vi "Keithley Sweep and Acquire Measurements.vi"(4 "Source Delay (s)":dbl=0.1, 5 "Sweep Direction":u16(ring) items=["Low to high", "High to low"], 6 "Number of Points":u32=5, 7 "Maximum Amplitude":dbl=2.0, 8 "Minimum Amplitude":dbl=1.0, 9 "VISA resource name":refnum<visa-resource-name>) -> (0 "Measurement Complete":bool, 2 "Data Array":dbl[][](array[numeric]), 3 "VISA resource name out":refnum<visa-resource-name>)   [LabVIEW 2011]
doc: "Configures a sweep and takes voltage and current readings at each point."
uses:
  <instrlib>/Keithley 24XX/Public/Data/Read (Multiple Points).vi
  <instrlib>/Keithley 24XX/Keithley 24XX.lvlib
panel:
  in  "Source Mode  (0: Voltage)":u16(ring) items=["Voltage", "Current"]
  in  "Timeout (10000 ms)":i32=60000 format="%#.6g"
  in  "Compliance  Level":dbl=0.1
  # "(c) 2006 National Instruments.  ALL RIGHTS RESERVED."
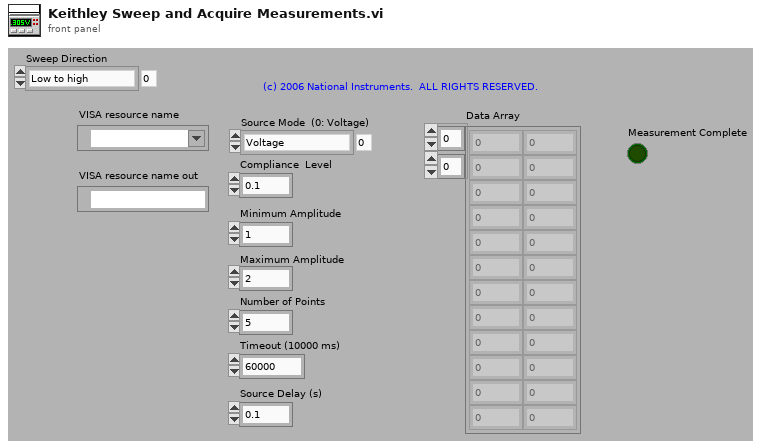
[diagram p1: front panel]
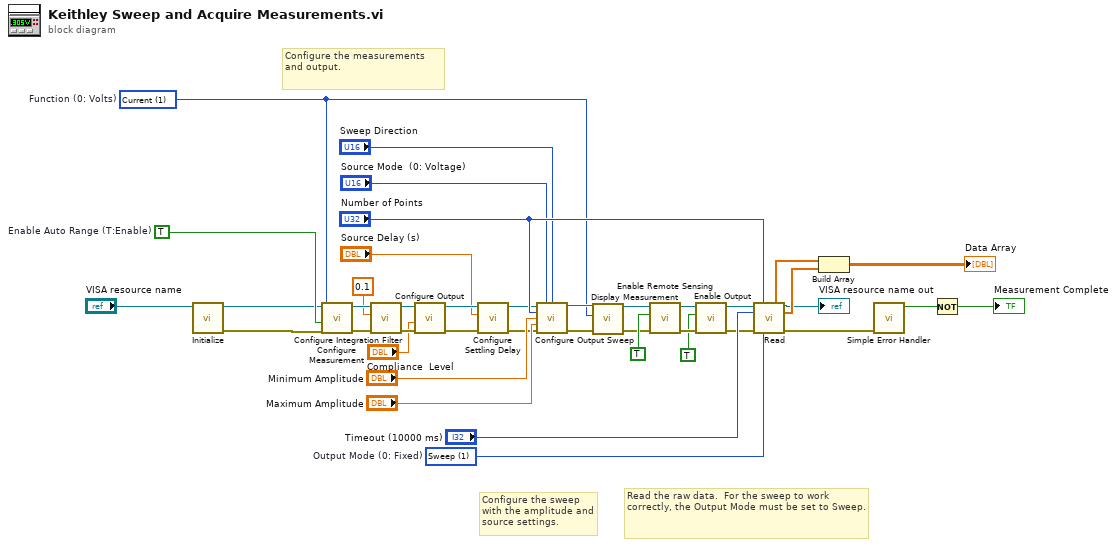
[diagram p0: block diagram]
diagram:
  w30 = TRUE  # Enable Auto Range (T:Enable)
  w12 = u16 1 items=["Volts", "Current", "Resistance"]  # Function (0: Volts)
  w33 = u16 1 items=["Fixed", "Sweep", "List"]  # Output Mode (0: Fixed)
  # "Read the raw data.  For the sweep to work correctly, the Output Mode must be set to Sweep."
  # "Configure the sweep with the amplitude and source settings."
  # "Configure the measurements and output."
  n1 = call <instrlib>:"Initialize.vi"("VISA resource name"="VISA resource name") -> ("error out"=w10:errorcluster, "VISA resource name out"=w11:refnum<visa-resource-name>)  [unwired: 9 in]
  n2 = call <instrlib>:"Configure Measurement.vi"("error in (no error)"=w10, "Enable Auto Range (T:Enable)"=w30, "Function (0: Volts)"=w12, "VISA resource name"=w11) -> ("error out"=w17:errorcluster, "VISA resource name out"=w18:refnum<visa-resource-name>)  [unwired: 6 in]
  n3 = call <instrlib>:"Configure Integration Filter.vi"("error in (no error)"=w17, "Measurement Speed (1 PLC)"=0.1, "VISA resource name"=w18) -> ("error out"=w8:errorcluster, "VISA resource name out"=w9:refnum<visa-resource-name>)  [unwired: 7 in]
  n4 = call <instrlib>:"Configure Output.vi"("error in (no error)"=w8, "Compliance  Level (0.1)"="Compliance  Level", "VISA resource name"=w9) -> ("error out"=w4:errorcluster, "VISA resource name out"=w5:refnum<visa-resource-name>)  [unwired: 7 in]
  n5 = call <instrlib>:"Configure Settling Delay.vi"("error in (no error)"=w4, "Manual Settling Delay (0 sec)"="Source Delay (s)", "VISA resource name"=w5) -> ("error out"=w2:errorcluster, "VISA resource name out"=w3:refnum<visa-resource-name>)  [unwired: 7 in]
  n6 = call <instrlib>:"Configure Output Sweep.vi"("VISA resource name"=w3, "Source Mode  (0: Voltage)"="Source Mode  (0: Voltage)", "Sweep Direction  (0: Ascending)"="Sweep Direction", "Number of Points (5)"="Number of Points", "Minimum Amplitude (1)"="Minimum Amplitude", "Maximum Amplitude (2)"="Maximum Amplitude", "error in (no error)"=w2) -> ("VISA resource name out"=w16:refnum<visa-resource-name>, "error out"=w15:errorcluster)  [unwired: 7 in]
  n7 = call <instrlib>:"Display Measurement.vi"("error in (no error)"=w15, "Displayed Measurement (0: Voltage)"=w12, "VISA resource name"=w16) -> ("error out"=w13:errorcluster, "VISA resource name out"=w14:refnum<visa-resource-name>)  [unwired: 7 in]
  n8 = call <instrlib>:"Enable Remote Sensing.vi"("error in (no error)"=w13, "Enable Remote Sensing (T: Enable)"=TRUE ("Enable Output (T: Enable)"), "VISA resource name"=w14) -> ("error out"=w22:errorcluster, "VISA resource name out"=w23:refnum<visa-resource-name>)  [unwired: 7 in]
  n9 = call <instrlib>:"Enable Output.vi"("error in (no error)"=w22, "Enable Output (T: Enable)"=TRUE, "VISA resource name"=w23) -> ("error out"=w32:errorcluster, "VISA resource name out"=w31:refnum<visa-resource-name>)  [unwired: 7 in]
  n10 = call-poly <instrlib>:"Read.vi"("VISA resource name"=w31, "Sample Count (1)"="Number of Points", "Timeout (10000 ms)"="Timeout (10000 ms)", "error in (no error)"=w32, "Output Mode (0: Fixed)"=w33) -> ("Voltage"=w37:sgl[], "VISA resource name out"=→"VISA resource name out":refnum<visa-resource-name>, "Current"=w36:sgl[], "error out"=w28:errorcluster)  [unwired: 4 in, 3 out]
  n11 = Build Array(w37, w36) -> (→"Data Array":sgl[][])
  n12 = call <vilib>:"Simple Error Handler.vi"("error in (no error)"=w28) -> ("error?"=w26:bool)  [unwired: 4 in, 4 out]
  n13 = Not(x=w26) -> (.not. x?=→"Measurement Complete":bool)
